vi "ds_Inner Part.vi"(5 "stopping criteria":T1={"function tolerance"=1e-06, "parameter tolerance"=1e-06, "max iterations"=0, "max function calls"=0, "gradient tolerance"=0.0, "max time (sec)"=1000.0, "initial tick count"=0}, 7 "function and data":T2, 8 "error in":errorcluster, 10 "f(Minimum) before":dbl[](array[numeric]) format="%.2f", 11 "Minimum before":dbl[][](array[numeric]) format="%.2f") -> (0 "error out":errorcluster, 1 "number of function evaluations":i32, 2 "f(Minimum) after":dbl[](array[numeric]) format="%.2f", 3 "Minimum after":dbl[][](array[numeric]) format="%.2f", 4 "convergence":bool)   [LabVIEW 2017, in "NI_Gmath.lvlib"]
uses:
  NI_Gmath.lvlib
  ucno_user function ref and data.ctl
  ucno_user objective function ref.ctl
  stopping criteria with time.ctl
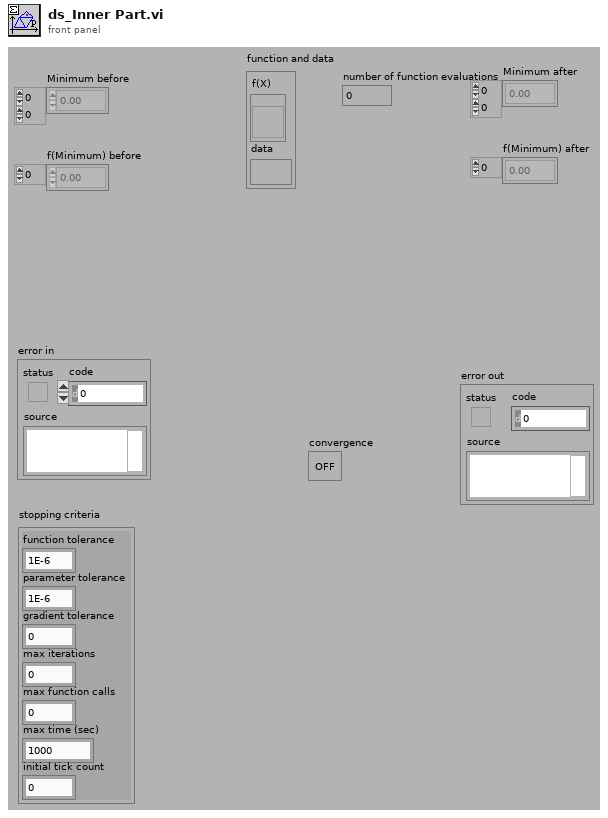
[diagram p1: front panel]
types:
  T1 = typedef "NI_Gmath.lvlib/stopping criteria with time.ctl" = cluster{"function tolerance":dbl, "parameter tolerance":dbl, "max iterations":i32, "max function calls":i32, "gradient tolerance":dbl, "max time (sec)":dbl, "initial tick count":u32}
  T2 = typedef "NI_Gmath.lvlib/ucno_user function ref and data.ctl" = cluster{"f(X)":T3, "data":variant}
  T3 = typedef "NI_Gmath.lvlib/ucno_user objective function ref.ctl" = refnum<vi>
  T4 = cluster{"objective function":bool, "gradient":bool}
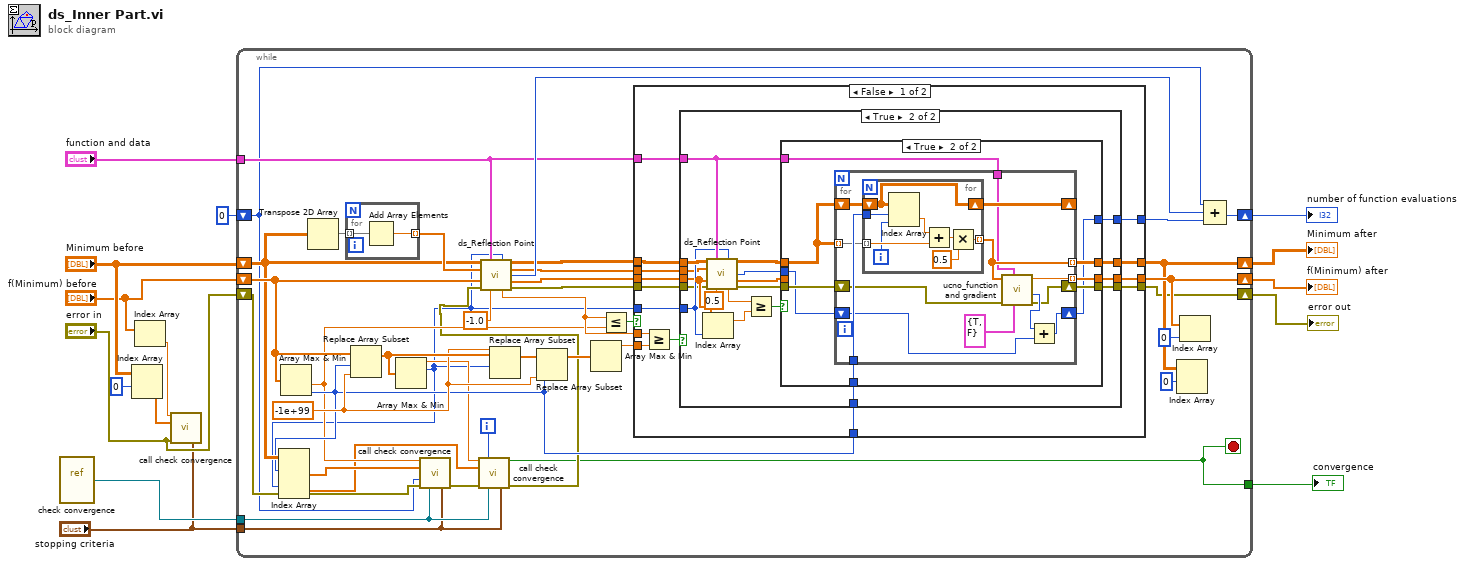
[diagram p0: block diagram]
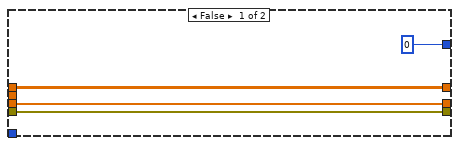
[diagram p2: hidden frame]
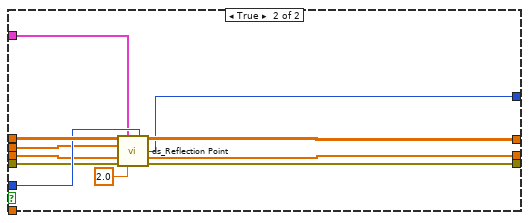
[diagram p4: hidden frame]
diagram:
  n1 = vi-ref "check convergence.vi"() -> ("vi reference"=w10:refnum<vi>)
  n2 = Index Array(array="Minimum before", index (row)=0) -> (element=w7:dbl[])  [unwired: 1 in]
  n3 = Index Array(array="f(Minimum) before") -> (element=w5:dbl)  [unwired: 1 in]
  n4 = call "call check convergence.vi"("f"=w5, "X"=w7, "error in"="error in", "stopping criteria"="stopping criteria") -> ()  [unwired: 7 in, 5 out]
  n5 = while {
    tunnel: [w19] -> w15
    shift-left: "f(Minimum) before" -> [w41]
    shift-right: [w37] -> w14
    shift-left: "Minimum before" -> [w33]
    shift-right: [w36] -> w13
    tunnel: "function and data" -> [w46]
    shift-right: [w23] -> w11
    shift-left: "error in" -> [w28]
    tunnel: w10 -> [w22]
    tunnel: "stopping criteria" -> [w21]
    shift-right: [w17] -> w1
    shift-left: 0 -> [w16]
    i -> [w20]
    stop <- w19 stop-if-true
    w38 = -1e+99
    n6 = Array Max & Min(array=w41) -> (min value=w30:dbl, min index (indices)=w32:i32)  [unwired: 2 out]
    n7 = Transpose 2D Array(2D array=w33) -> (transposed array=w53:dbl[][])
    n8 = for {
      tunnel: w53 -> [w138] mode=indexing
      tunnel: [w137] -> w43 mode=indexing
      n9 = Add Array Elements(numeric array=w138) -> (sum=w137:dbl)
    }
    n10 = Replace Array Subset(array=w41, new element=w38, index=w32) -> (w47:dbl[])
    n11 = Array Max & Min(array=w47) -> (max value=w26:dbl, max index (indices)=w25:i32)  [unwired: 2 out]
    n12 = Index Array(array=w33, index (row) #1=w32, index (row) #2=w25) -> (element #1=w31:dbl[], element #2=w24:dbl[])  [unwired: 2 in]
    n13 = call "call check convergence.vi"("f"=w30, "X"=w31, "number of function evaluations"=w16, "error in"=w28, "vi reference"=w22, "stopping criteria"=w21) -> ("error out"=w29:errorcluster)  [unwired: 5 in, 4 out]
    n14 = call "call check convergence.vi"("f"=w26, "current iteration"=w20, "X"=w24, "error in"=w29, "vi reference"=w22, "stopping criteria"=w21) -> ("stop?"=w19:bool, "error out"=w27:errorcluster)  [unwired: 5 in, 3 out]
    n15 = call "ds_Reflection Point.vi"("points before"=w33, "function and data"=w46, "high index"=w25, "psum before"=w43, "f values before"=w41, "error in (no error)"=w27, "factor"=-1.0) -> ("points after"=w51:dbl[][], "psum after"=w42:dbl[], "number of function calls"=w54:i32, "f values after"=w40:dbl[], "new f value"=w45:dbl, "error out"=w39:errorcluster)  [unwired: 3 in]
    n16 = Replace Array Subset(array=w47, new element=w38, index=w25) -> (w49:dbl[])
    n17 = Replace Array Subset(array=w49, new element=w38, index=w32) -> (w48:dbl[])
    n18 = Array Max & Min(array=w48) -> (max value=w50:dbl)  [unwired: 3 out]
    n19 = Less Or Equal?(x=w45, y=w30) -> (x <= y?=w52:bool)
    n20 = case shown="False" w52 {
      tunnel: w51 -> [w65 w136]
      tunnel: w42 -> [w64 w132]
      tunnel: w40 -> [w59 w131]
      tunnel: w25 -> [w63 w134]
      tunnel: [w61 w135] -> w36
      tunnel: [w60 w130] -> w37
      tunnel: w45 -> [w68 _]
      tunnel: w50 -> [w67 _]
      tunnel: w32 -> [w62 _]
      tunnel: w46 -> [w58 w126]
      tunnel: w39 -> [w57 w128]
      tunnel: [w56 w129] -> w23
      tunnel: [w55 w127] -> w18
      frame False {
        n21 = Greater Or Equal?(x=w68, y=w67) -> (x >= y?=w66:bool)
        n22 = case shown="True" w66 {
          tunnel: w65 -> [w72 w91]
          tunnel: w64 -> [_ w80]
          tunnel: w59 -> [w71 w79]
          tunnel: w63 -> [_ w83]
          tunnel: w62 -> [_ w89]
          tunnel: [w72 w87] -> w61
          tunnel: [w71 w86] -> w60
          tunnel: w58 -> [_ w84]
          tunnel: w57 -> [w70 w77]
          tunnel: [w70 w75] -> w56
          tunnel: [0 ("number of function calls") w73] -> w55
          frame False {
          }
          frame True {
            n23 = Index Array(array=w79, index=w83) -> (element=w85:dbl)
            n24 = call "ds_Reflection Point.vi"("points before"=w91, "function and data"=w84, "high index"=w83, "psum before"=w80, "f values before"=w79, "error in (no error)"=w77, "factor"=0.5) -> ("points after"=w88:dbl[][], "number of function calls"=w74:i32, "f values after"=w78:dbl[], "new f value"=w81:dbl, "error out"=w76:errorcluster)  [unwired: 3 in, 1 out]
            n25 = Greater Or Equal?(x=w81, y=w85) -> (x >= y?=w90:bool)
            n26 = case shown="True" w90 {
              tunnel: w89 -> [_ w104]
              tunnel: w88 -> [w95 w101]
              tunnel: [w95 w103] -> w87
              tunnel: [w94 w102] -> w86
              tunnel: w78 -> [w94 _]
              tunnel: w84 -> [_ w100]
              tunnel: w76 -> [w93 w99]
              tunnel: [w93 w98] -> w75
              tunnel: w74 -> [w92 w97]
              tunnel: [w92 w96] -> w73
              frame False {
              }
              frame True {
                n27 = for {
                  tunnel: w104 -> [w114]
                  shift-right: [w115] -> _
                  shift-left: w101 -> [w116]
                  tunnel: w101 -> [w113] mode=indexing
                  tunnel: [w112] -> w103 mode=indexing
                  tunnel: [w111] -> w102 mode=indexing
                  tunnel: w100 -> [w108]
                  shift-right: [w109] -> w98
                  shift-left: w99 -> [w110]
                  shift-right: [w106] -> w96
                  shift-left: w97 -> [w105]
                  n28 = for {
                    shift-right: [w120] -> w115
                    shift-left: w116 -> [w120]
                    tunnel: w114 -> [w118]
                    tunnel: w113 -> [w125] mode=indexing
                    tunnel: [w121] -> w112 mode=indexing
                    i -> [w119]
                    n29 = Index Array(array=w120, index (row)=w118, index (col)=w119) -> (element=w124:dbl)
                    n30 = Add(x=w124, y=w125) -> (x+y=w123:dbl)
                    n31 = Multiply(x=w123, y=0.5) -> (x*y=w121:dbl)
                  }
                  n32 = call "ucno_function and gradient.vi"("output control"=T4 {"objective function"=TRUE, "gradient"=FALSE}, "function and data"=w108, "error in (no error)"=w110, "X"=w112) -> ("error out"=w109:errorcluster, "number of function calls"=w117:i32, "f(X)"=w111:dbl)  [unwired: 4 in, 1 out]
                  n33 = Add(x=w117, y=w105) -> (x+y=w106:i32)
                }
              }
            }
          }
        }
      }
      frame True {
        n34 = call "ds_Reflection Point.vi"("points before"=w136, "function and data"=w126, "high index"=w134, "psum before"=w132, "f values before"=w131, "error in (no error)"=w128, "factor"=2.0) -> ("points after"=w135:dbl[][], "number of function calls"=w127:i32, "f values after"=w130:dbl[], "error out"=w129:errorcluster)  [unwired: 3 in, 2 out]
      }
    }
    n35 = Index Array(array=w36, index (row)=0) -> ()  [unwired: 1 in, 1 out]
    n36 = Index Array(array=w37, index=0) -> ()  [unwired: 1 out]
    n37 = Compound Arithmetic op=ADD(w16, w54, w18) -> (w17:i32)
  }
  "convergence" <- w15
  "f(Minimum) after" <- w14
  "Minimum after" <- w13
  "error out" <- w11
  "number of function evaluations" <- w1
